vi "GetLocalConfiguration.vi"() -> (1 "Configuration File":path)   [LabVIEW 2018]
uses:
  globals/QC_RunInformation.vi
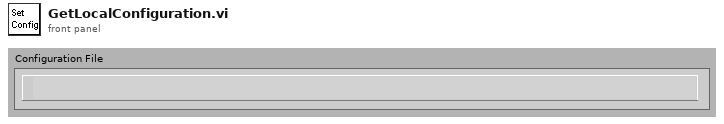
[diagram p1: front panel]
types:
  T1 = cluster{"Institute":string, "Manufacturers":string[], "Devices":string[], "Serialnumbers Lookup DB":string, "Data directory":string, "Backup & screenshot directory":string, "List of known users":string[], "Measurement switch not used":bool, "Measurement Switch":string, "DUT Switch":string, "Rseries IV [MOhm]":string, "Rshunt IV [MOhm]":string, "Rseries CV [MOhm]":string, "DC blocking Cap [µF]":string, "Rseries LCR [MOhm]":string, "Rseries stability [MOhm]":string, "Rshunt stability [MOhm]":string, "Rseries striptest bias [MOhm]":string, "Rseries strip pinhole [MOhm]":string}
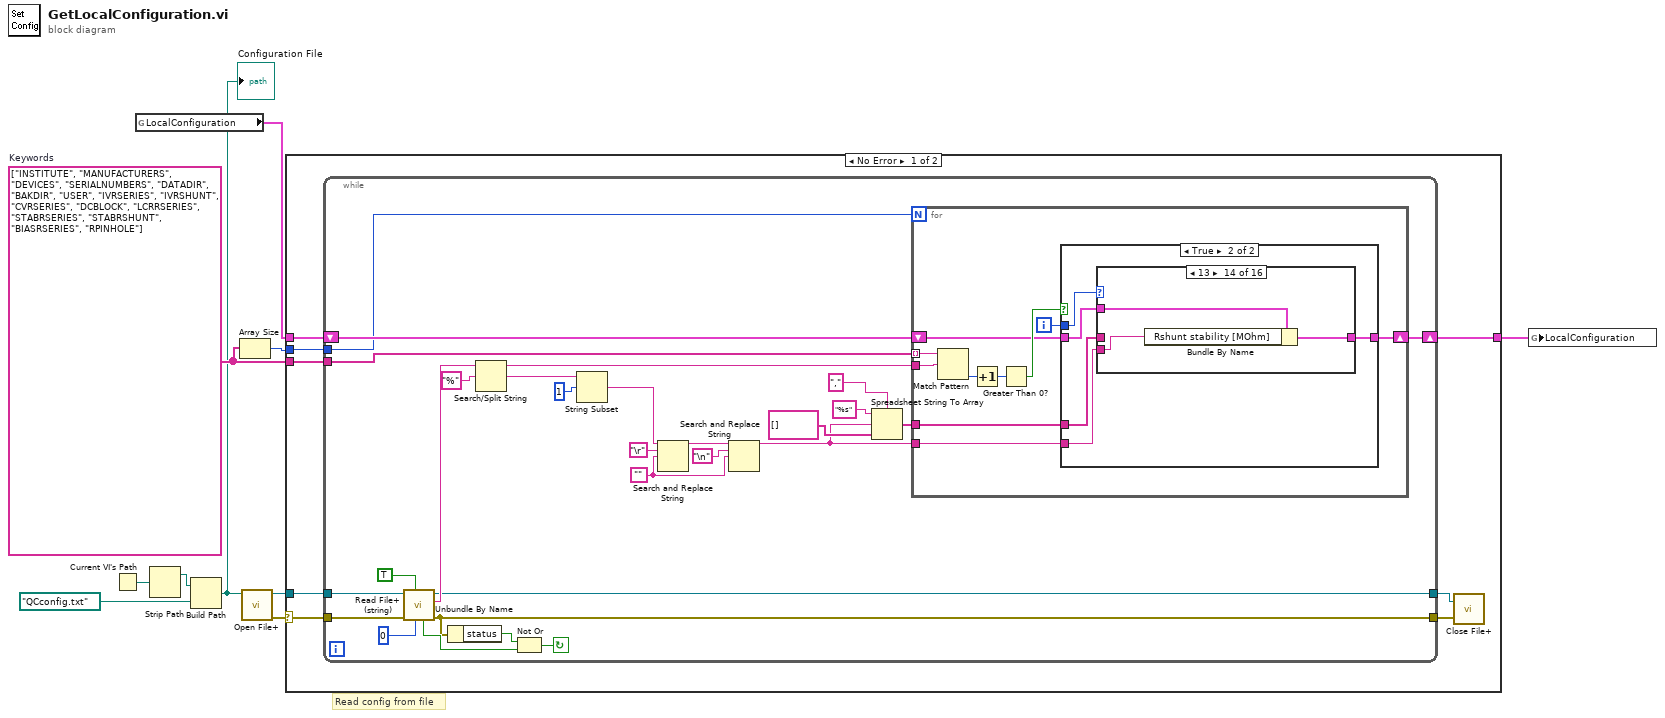
[diagram p0: block diagram]
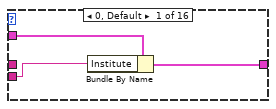
[diagram p3: hidden frame]
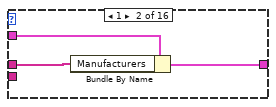
[diagram p4: hidden frame]
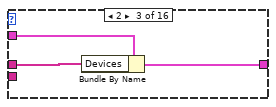
[diagram p5: hidden frame]
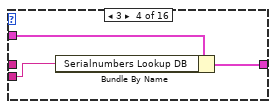
[diagram p6: hidden frame]
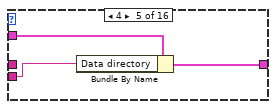
[diagram p7: hidden frame]
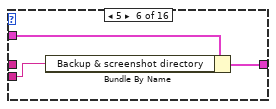
[diagram p8: hidden frame]
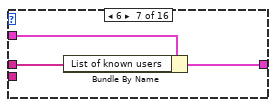
[diagram p9: hidden frame]
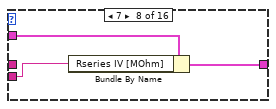
[diagram p10: hidden frame]
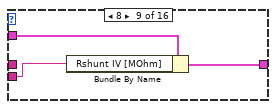
[diagram p11: hidden frame]
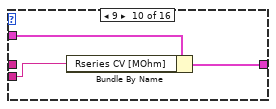
[diagram p12: hidden frame]
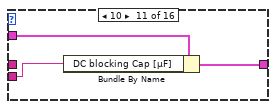
[diagram p13: hidden frame]
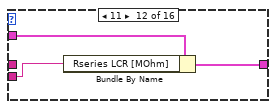
[diagram p14: hidden frame]
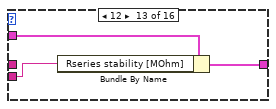
[diagram p15: hidden frame]
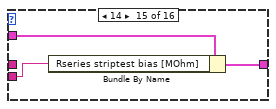
[diagram p16: hidden frame]
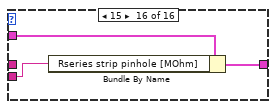
[diagram p17: hidden frame]
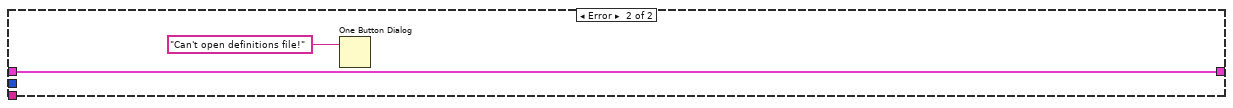
[diagram p18: hidden frame]
diagram:
  w10 = string[] ["INSTITUTE", "MANUFACTURERS", "DEVICES", "SERIALNUMBERS", "DATADIR", "BAKDIR", "USER", "IVRSERIES", "IVRSHUNT", "CVRSERIES", "DCBLOCK", "LCRRSERIES", "STABRSERIES", "STABRSHUNT", "BIASRSERIES", "RPINHOLE"]  # Keywords
  # "Read config from file"
  n1 = Current VI's Path() -> (path=w3:path)
  n2 = global read "QC_RunInformation.vi" "LocalConfiguration"() -> (w8:T1)
  n3 = Strip Path(path=w3) -> (stripped path=w2:path)  [unwired: 1 out]
  n4 = Build Path(base path=w2, name or relative path=path "QCconfig.txt") -> (appended path=w1:path)
  "Configuration File" <- w1
  n5 = Array Size(array=w10) -> (size(s)=w9:i32)
  n6 = call <vilib>:"Open File+.vi"("file path (\" \")"=w1) -> ("error out"=w4:errorcluster, "refnum"=w5:refnum<file>)  [unwired: 7 in, 2 out]
  n7 = case shown="No Error" w4 {
    selector: w4 -> [w11 _]
    tunnel: w5 -> [w18 _]
    tunnel: w10 -> [w17 _]
    tunnel: w9 -> [w16 _]
    tunnel: w8 -> [w15 w111]
    tunnel: [w14 w111] -> w6
    frame No Error {
      n8 = while {
        shift-left: w15 -> [w27]
        shift-right: [w26] -> w14
        tunnel: w16 -> [w25]
        tunnel: w17 -> [w30]
        tunnel: [w32] -> w12
        tunnel: w11 -> [w33]
        tunnel: [w34] -> w13
        tunnel: w18 -> [w40]
        stop <- w36 continue-if-true
        w22 = ""
        n9 = call <vilib>:"Read File+ (string).vi"("count"=0, "line mode (characters:F)"=TRUE, "error in (no error)"=w33, "refnum"=w40) -> ("error out"=w32:errorcluster, "string"=w35:string, "dup refnum"=w34:refnum<file>, "EOF?"=w38:bool)  [unwired: 3 in, 1 out]
        n10 = Unbundle By Name(w32) -> ("status"=w37:bool)
        n11 = Search/Split String(string=w35, search string/char (-)="%" ("search char (-)")) -> (substring before match=w29:string, match + rest of string=w42:string)  [unwired: 1 in, 1 out]
        n12 = Not Or(1:w38, 2:w37) -> (0:w36:bool)
        n13 = String Subset(string=w42, offset (0)=1) -> (substring=w20:string)  [unwired: 1 in]
        n14 = Search and Replace String(input string=w20, search string="\r", replace string=w22) -> (result string=w21:string)  [unwired: 5 in, 3 out]
        n15 = Search and Replace String(input string=w21, search string="\n", replace string=w22) -> (result string=w19:string)  [unwired: 5 in, 3 out]
        n16 = Spreadsheet String To Array(delimiter (Tab)=",", format string="%s", spreadsheet string=w19, array type (2D Dbl)=string[] []) -> (array=w28:string[])
        n17 = for {
          N: w25 -> [_]
          tunnel: w30 -> [w54] mode=indexing
          tunnel: w29 -> [w48]
          tunnel: w28 -> [w51]
          shift-right: [w49] -> w26
          shift-left: w27 -> [w50]
          tunnel: w19 -> [w47]
          i -> [w52]
          n18 = Match Pattern(string=w54, regular expression=w48) -> (offset past match=w55:i32)  [unwired: 1 in, 3 out]
          n19 = Increment(x=w55) -> (x+1=w56:i32)
          n20 = Greater Than 0?(x=w56) -> (x > 0?=w53:bool)
          n21 = case shown="True" w53 {
            tunnel: w52 -> [_ w62]
            tunnel: w51 -> [_ w61]
            tunnel: w47 -> [_ w60]
            tunnel: w50 -> [w57 w59]
            tunnel: [w57 w58] -> w49
            frame False {
            }
            frame True {
              n22 = case shown="13" w62 {
                tunnel: w61 -> [_ w67 w70 _ _ _ w81 _ _ _ _ _ _ _ _ _]
                tunnel: w60 -> [w63 _ _ w72 w75 w78 _ w84 w87 w90 w93 w96 w99 w102 w105 w108]
                tunnel: w59 -> [w65 w68 w71 w74 w77 w80 w83 w86 w89 w92 w95 w98 w101 w104 w107 w110]
                tunnel: [w64 w66 w69 w73 w76 w79 w82 w85 w88 w91 w94 w97 w100 w103 w106 w109] -> w58
                frame 0, Default {
                  n23 = Bundle By Name(cluster=w65, "Institute"=w63) -> (w64:T1)
                }
                frame 1 {
                  n24 = Bundle By Name(cluster=w68, "Manufacturers"=w67) -> (w66:T1)
                }
                frame 2 {
                  n25 = Bundle By Name(cluster=w71, "Devices"=w70) -> (w69:T1)
                }
                frame 3 {
                  n26 = Bundle By Name(cluster=w74, "Serialnumbers Lookup DB"=w72) -> (w73:T1)
                }
                frame 4 {
                  n27 = Bundle By Name(cluster=w77, "Data directory"=w75) -> (w76:T1)
                }
                frame 5 {
                  n28 = Bundle By Name(cluster=w80, "Backup & screenshot directory"=w78) -> (w79:T1)
                }
                frame 6 {
                  n29 = Bundle By Name(cluster=w83, "List of known users"=w81) -> (w82:T1)
                }
                frame 7 {
                  n30 = Bundle By Name(cluster=w86, "Rseries IV [MOhm]"=w84) -> (w85:T1)
                }
                frame 8 {
                  n31 = Bundle By Name(cluster=w89, "Rshunt IV [MOhm]"=w87) -> (w88:T1)
                }
                frame 9 {
                  n32 = Bundle By Name(cluster=w92, "Rseries CV [MOhm]"=w90) -> (w91:T1)
                }
                frame 10 {
                  n33 = Bundle By Name(cluster=w95, "DC blocking Cap [µF]"=w93) -> (w94:T1)
                }
                frame 11 {
                  n34 = Bundle By Name(cluster=w98, "Rseries LCR [MOhm]"=w96) -> (w97:T1)
                }
                frame 12 {
                  n35 = Bundle By Name(cluster=w101, "Rseries stability [MOhm]"=w99) -> (w100:T1)
                }
                frame 13 {
                  n36 = Bundle By Name(cluster=w104, "Rshunt stability [MOhm]"=w102) -> (w103:T1)
                }
                frame 14 {
                  n37 = Bundle By Name(cluster=w107, "Rseries striptest bias [MOhm]"=w105) -> (w106:T1)
                }
                frame 15 {
                  n38 = Bundle By Name(cluster=w110, "Rseries strip pinhole [MOhm]"=w108) -> (w109:T1)
                }
              }
            }
          }
        }
      }
      n39 = call <vilib>:"Close File+.vi"("error in (no error)"=w12, "refnum"=w13) -> ()  [unwired: 3 in, 3 out]
    }
    frame Error {
      n40 = One Button Dialog(message="Can't open definitions file!") -> ()  [unwired: 1 in, 1 out]
    }
  }
  n41 = global write "QC_RunInformation.vi" "LocalConfiguration"(w6) -> ()
